vi "GetAnalysisBdcstEvents.vi"(7 "error in (no error)":errorcluster) -> (3 "Event Registration Refnum":refnum<event-registration>, 5 "error out":errorcluster)   [LabVIEW 2018, in "Test.lvclass"]
uses:
  Test.lvclass
  Analysis/AnalysisModule/Protected/clEventType.ctl
  Analysis/AnalysisModule/AnalysisModule.lvlib
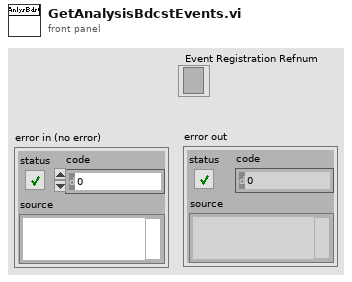
[diagram p1: front panel]
types:
  T1 = typedef "AnalysisModule.lvlib/clBroadcastEvents.ctl" = cluster{"DidInit":refnum<user-event>, "StatusUpdate":refnum<user-event>, "ErrorReport":refnum<user-event>, "DidStop":refnum<user-event>, "PathToINI":refnum<user-event>, "Config":refnum<user-event>, "ResultReport":refnum<user-event>, "FunctionClass":refnum<user-event>, "State":refnum<user-event>, "FunctionParams":refnum<user-event>, "Duration":refnum<user-event>}
  T2 = cluster{"State":refnum<user-event>, "FunctionClass":refnum<user-event>, "ErrorReport":refnum<user-event>, "Config":refnum<user-event>, "Duration":refnum<user-event>}
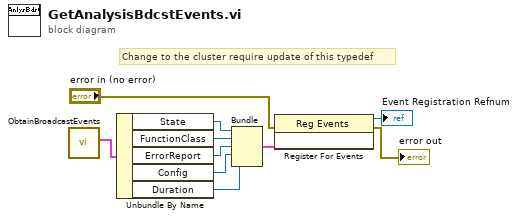
[diagram p0: block diagram]
diagram:
  # "Change to the cluster require update of this typedef"
  n1 = call "ObtainBroadcastEvents.vi"() -> ("clBroadcastEvents"=w10:T1)  [unwired: 10 in, 1 out]
  n2 = Unbundle By Name(w10) -> ("State"=w6:refnum<user-event>, "FunctionClass"=w9:refnum<user-event>, "ErrorReport"=w8:refnum<user-event>, "Config"=w3:refnum<user-event>, "Duration"=w2:refnum<user-event>)
  n3 = Bundle("State"=w6, "FunctionClass"=w9, "ErrorReport"=w8, "Config"=w3, "Duration"=w2) -> (w7:T2)  [unwired: 1 in]
  n4 = register-events(error in="error in (no error)", w7) -> (reference out=→"Event Registration Refnum":refnum<event-registration>, error out=→"error out":errorcluster)  [unwired: 1 in]
